vi "GV DO2.vi"() -> ()   [LabVIEW 2017]
panel:
  out "DO2":bool
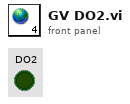
[diagram p1: front panel]
diagram:
